vi "Is Connected.vi"(8 "error in (no error)":errorcluster, 11 "VISA Stream in":refnum<class "Serial Stream.lvclass">) -> (0 "error out":errorcluster, 2 "Connected":bool, 3 "VISA Stream out":refnum<class "Serial Stream.lvclass">)   [LabVIEW 2020, in "Stream-Serial.lvlib" / "Serial Stream.lvclass"]
uses:
  Serial Stream.lvclass
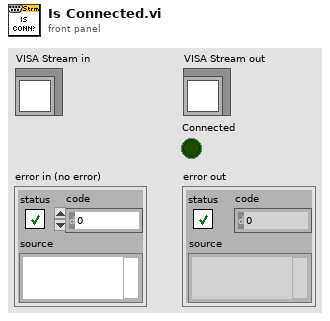
[diagram p1: front panel]
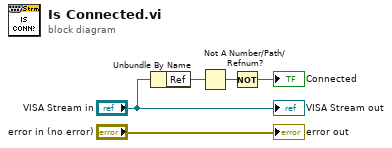
[diagram p0: block diagram]
diagram:
  n1 = Unbundle By Name("VISA Stream in") -> ("Ref"=w3:refnum<data-value>)
  n2 = Not A Number/Path/Refnum?(number/path/refnum=w3) -> (NaN/Path/Refnum?=w2:bool)
  n3 = Not(x=w2) -> (.not. x?=→"Connected":bool)
  "error out" <- "error in (no error)"
  "VISA Stream out" <- "VISA Stream in"
